vi "Write Spectral Calibration.vi"(8 "Central WL":dbl[unit], 9 "Central Pixel":i32, 10 "nm per px":dbl[unit], 11 "Analyze Parameter Spectral Calibration in":refnum<class "Analyze Parameter Spectral Calibration.lvclass">) -> (3 "Analyze Parameter Spectral Calibration out":refnum<class "Analyze Parameter Spectral Calibration.lvclass">)   [LabVIEW 2014, in "Analyze Parameter Spectral Calibration.lvclass"]
uses:
  Analyze Parameter Spectral Calibration.lvclass
  Analyze Parameter Spectral Calibration.lvclass/Analyze Parameter Spectral Calibration.ctl
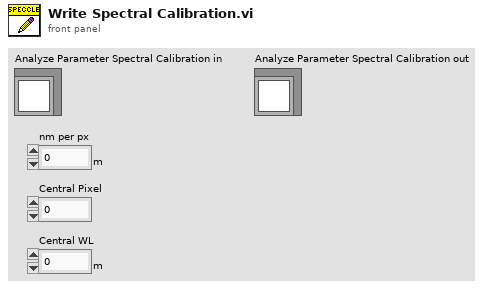
[diagram p1: front panel]
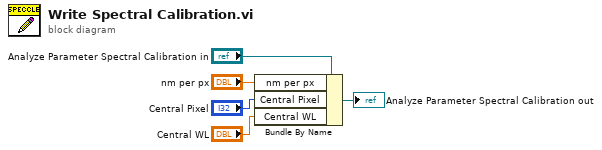
[diagram p0: block diagram]
diagram:
  n1 = Bundle By Name(cluster="Analyze Parameter Spectral Calibration in", "nm per px"="nm per px", "Central Pixel"="Central Pixel", "Central WL"="Central WL") -> (→"Analyze Parameter Spectral Calibration out":refnum<class "Analyze Parameter Spectral Calibration.lvclass">)
